vi "bulk_read_write.vi"() -> ()   [LabVIEW 2022 SP3]
uses:
  Library/dxl_x64_c.lvlib
panel:
  out "dynamixel_error":string
  out "dynamixel_comm_result":string
  in  "value : PRO (slide)\nLED RED":bool
  in  "LEN_PRO_\nGOAL_POSITION":u16=4
  out "groupwrite_num":i32
  in  "LEN_PRO_\nLED_RED":u16=1
  in  "ADDR_PRO_\nLED_RED":u16=563
  out "value : PRO (LED)\nLED_RED":bool
  out "groupread_num":i32
  in  "LEN_PRO_\nPRESENT_POSITION":u16=4
  in  "dynamixe2_id":u8=2
  in  "device_name":string="COM1"
  in  "ADDR_PRO_\nPRESENT_POSITION":u16=611
  in  "ADDR_PRO_\nGOAL_POSITION":u16=596
  in  "ADDR_PRO_\nTORQUE_ENABLE":u16=562
  out "protocol_version":dbl=2.0
  out "value : PRO (knob)\npresent position 1":i32(knob) scale=150000.0..-150000.0
  in  "terminate":bool
  out "port_num":i32
  in  "value : PRO (dial)\ngoal position":i32(knob) scale=150000.0..-150000.0
  in  "dynamixel1_id":u8=1
  in  "baud_rate":i32=57600
  # "/*******************************************************************************\n* Copyright (c) 2016, ROBOTIS CO., LTD.\n* All rights reserved.\n*\n* Redistribution and use in source and binary forms, with or without\n* modification, are permitted provided that the following conditions are met:\n*\n* * Redistributions of source code must retain the above copyright notice, this\n*   list of conditions and the following disclaimer.\n*\n* * Redistributions in binary form must reproduce the above copyright notice,\n*   this list of conditions and the following disclaimer in the documentation\n*   and/or other materials provided with the distribution.\n*\n* * Neither the name of ROBOTIS nor the names of its\n*   contributors may be used to endorse or promote products derived from\n*   this software without specific prior written permission.\n*\n* THIS SOFTWARE IS PROVIDED BY THE COPYRIGHT HOLDERS AND CONTRIBUTORS \"AS IS\"\n* AND ANY EXPRESS OR IMPLIED WARRANTIES, INCLUDING, BUT NOT LIMITED TO, THE\n* IMPLIED WARRANTIES OF MERCHANTABILITY AND FITNESS FOR A PARTICULAR PURPOSE ARE\n* DISCLAIMED. IN NO EVENT SHALL THE COPYRIGHT HOLDER OR CONTRIBUTORS BE LIABLE\n* FOR ANY DIRECT, INDIRECT, INCIDENTAL, SPECIAL, EXEMPLARY, OR CONSEQUENTIAL\n* DAMAGES (INCLUDING, BUT NOT LIMITED TO, PROCUREMENT OF SUBSTITUTE GOODS OR\n* SERVICES; LOSS OF USE, DATA, OR PROFITS; OR BUSINESS INTERRUPTION) HOWEVER\n* CAUSED AND ON ANY THEORY OF LIABILITY, WHETHER IN CONTRACT, STRICT LIABILITY,\n* OR TORT (INCLUDING NEGLIGENCE OR OTHERWISE) ARISING IN ANY WAY OUT OF THE USE\n* OF THIS SOFTWARE, EVEN IF ADVISED OF THE POSSIBILITY OF SUCH DAMAGE.\n*******************************************************************************/\n\n/* Author: Ryu Woon Jung (Leon) */"
  # "Available Dynamixel model on this example : All models using Protocol 2.0\nThis example is designed for using two Dynamixel PRO 54-200, and an USB2DYNAMIXEL.\nTo use another Dynamixel model, such as X series, see their details in E-Manual(support.robotis.com) \n   and edit \"numeric control\"s seen left with \"Edit Text\" tool.\nBe sure that Dynamixel PRO properties are already set as %% ID : 1 / Baudnum : 1 (Baudrate : 57600)\n\n1. Run example by click above \"Run\" button (below \"Edit\" menu).\n2. Drag \"dial\" then you may see the Dynamixel and \"knob\"s rotating\n3. Click \"slide button\" then you may see the LED of Dynamixel lighting\n4. To finish the example, press \"terminate\" button."
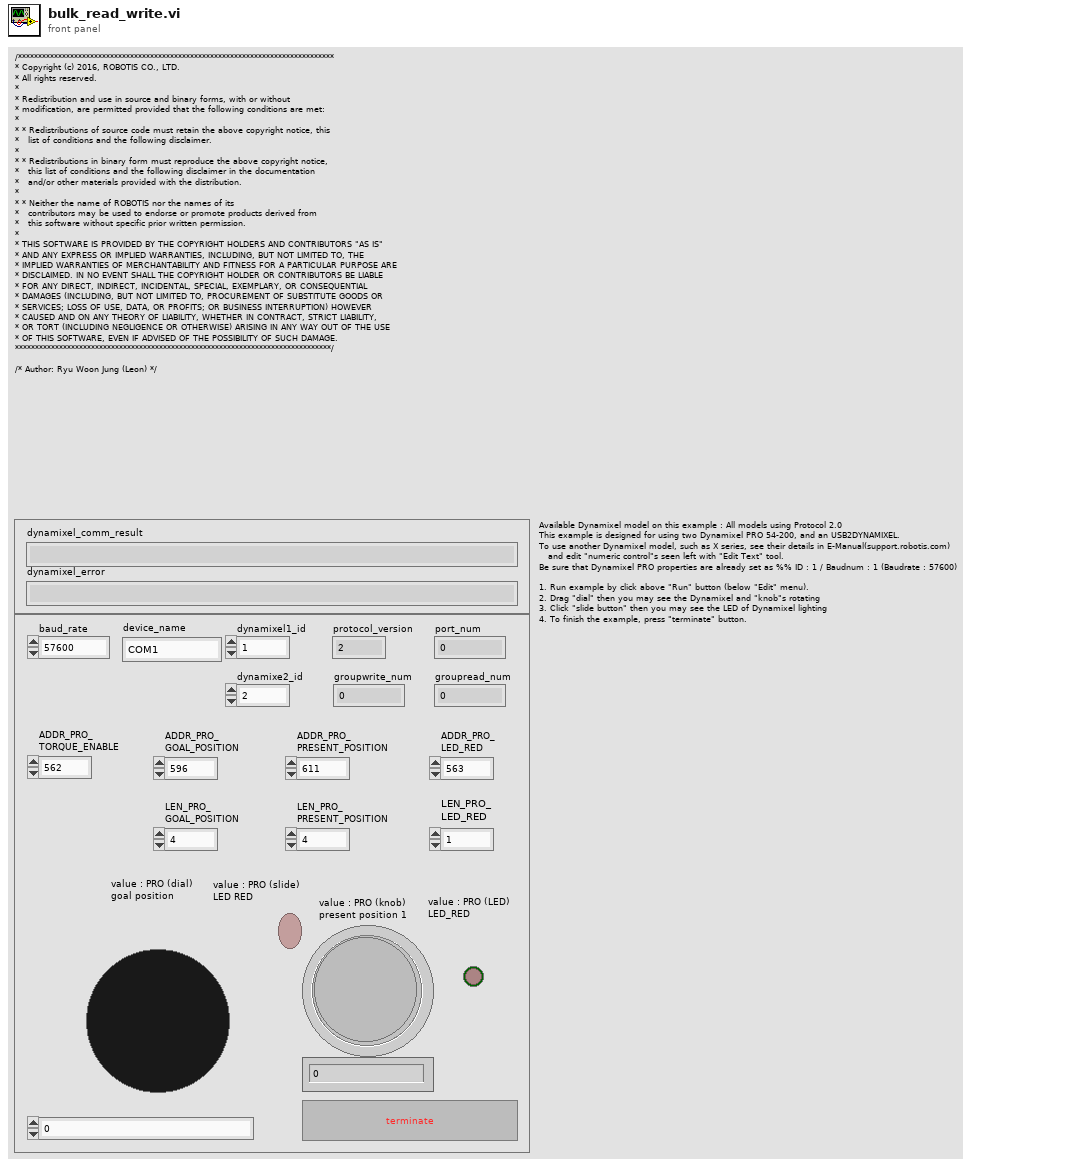
[diagram p1: front panel]
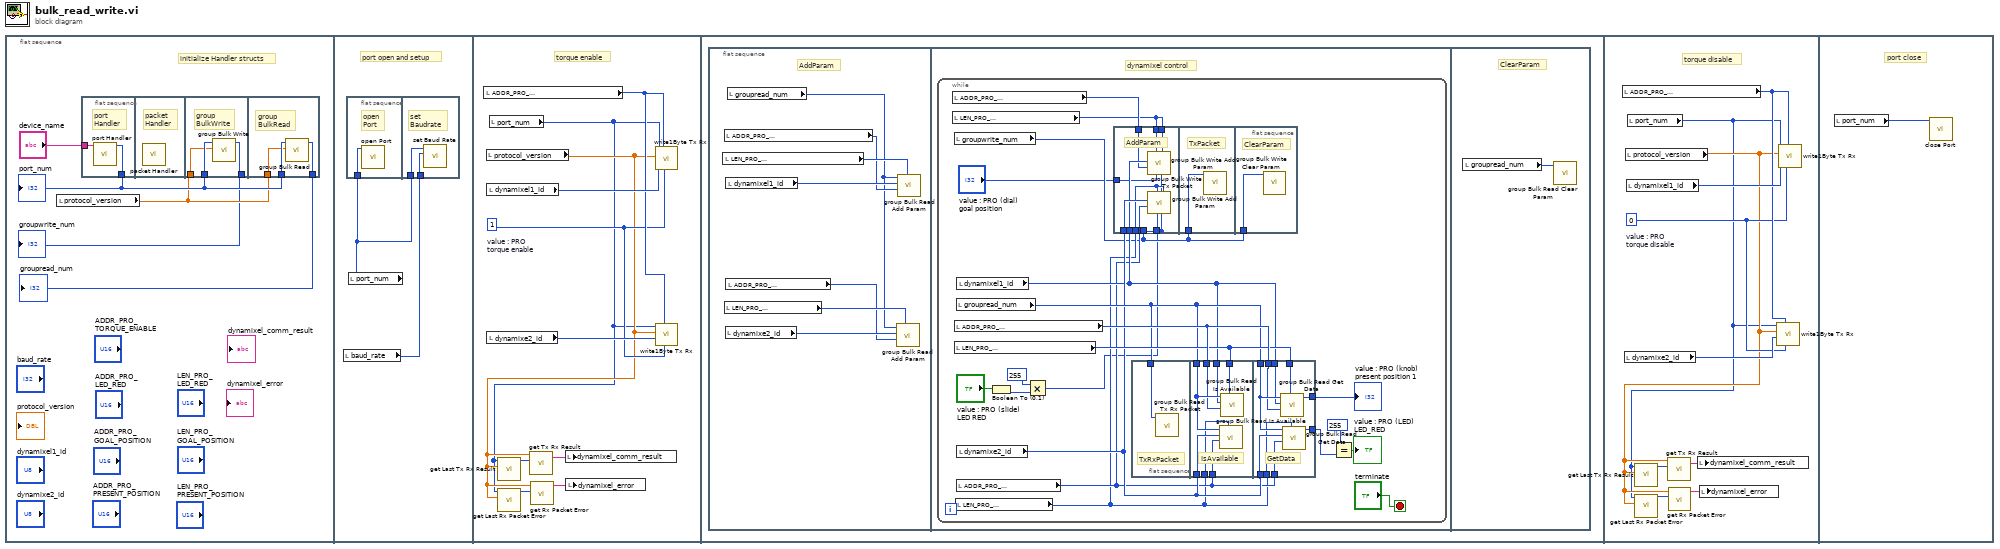
[diagram p0: block diagram]
diagram:
  n1 = flat-sequence {
    frame #0 {
      # "initialize Handler structs"
      n2 = local read "protocol_version"() -> (w3:dbl)
      n3 = flat-sequence {
        tunnel: "device_name" -> [w7]
        tunnel: [w6] -> w4
        tunnel: w3 -> [w8]
        tunnel: w4 -> [w10]
        tunnel: [w9] -> w2
        tunnel: w4 -> [w13]
        tunnel: w3 -> [w12]
        tunnel: [w11] -> w1
        frame #0 {
          # "port\nHandler"
          n4 = call "port Handler.vi"("port_name"=w7) -> ("function return"=w6:i32)  [unwired: 9 in, 1 out]
        }
        frame #1 {
          # "packet\nHandler"
          n5 = call "packet Handler.vi"() -> ()  [unwired: 11 in, 1 out]
        }
        frame #2 {
          # "group\nBulkWrite"
          n6 = call "group Bulk Write.vi"("protocol_version"=w8, "port_num"=w10) -> ("function return"=w9:i32)  [unwired: 8 in, 1 out]
        }
        frame #3 {
          # "group\nBulkRead"
          n7 = call "group Bulk Read.vi"("protocol_version"=w12, "port_num"=w13) -> ("function return"=w11:i32)  [unwired: 8 in, 1 out]
        }
      }
      "port_num" <- w4
      "groupread_num" <- w1
      "groupwrite_num" <- w2
    }
    frame #1 {
      # "port open and setup"
      n8 = local read "baud_rate"() -> (w14:i32)
      n9 = flat-sequence {
        tunnel: w15 -> [w16]
        tunnel: w15 -> [w18]
        tunnel: w14 -> [w17]
        frame #0 {
          # "open\nPort"
          n10 = call "open Port.vi"("port_num"=w16) -> ()  [unwired: 9 in, 2 out]
        }
        frame #1 {
          # "set\nBaudrate"
          n11 = call "set Baud Rate.vi"("baudrate"=w17, "port_num"=w18) -> ()  [unwired: 8 in, 2 out]
        }
      }
      n12 = local read "port_num"() -> (w15:i32)
    }
    frame #2 {
      w25 = 1  # value : PRO torque enable
      # "torque enable"
      n13 = local read "ADDR_PRO_\nTORQUE_ENABLE"() -> (w27:u16)
      n14 = local read "protocol_version"() -> (w20:dbl)
      n15 = local read "dynamixel1_id"() -> (w28:u8)
      n16 = local read "dynamixe2_id"() -> (w26:u8)
      n17 = local read "port_num"() -> (w19:i32)
      n18 = call "get Last Tx Rx Result.vi"("protocol_version"=w20, "port_num"=w19) -> ("function return"=w21:i32)  [unwired: 8 in, 1 out]
      n19 = call "get Last Rx Packet Error.vi"("protocol_version"=w20, "port_num"=w19) -> ("function return"=w22:u8)  [unwired: 8 in, 1 out]
      n20 = call "get Tx Rx Result.vi"("result"=w21, "protocol_version"=w20) -> ("function return"=w24:string)  [unwired: 8 in, 1 out]
      n21 = call "get Rx Packet Error.vi"("error"=w22, "protocol_version"=w20) -> ("function return"=w23:string)  [unwired: 8 in, 1 out]
      n22 = local write "dynamixel_comm_result"(w24) -> ()
      n23 = local write "dynamixel_error"(w23) -> ()
      n24 = call "write1Byte Tx Rx.vi"("data"=w25, "address"=w27, "id"=w28, "protocol_version"=w20, "port_num"=w19) -> ()  [unwired: 6 in, 1 out]
      n25 = call "write1Byte Tx Rx.vi"("data"=w25, "address"=w27, "id"=w26, "protocol_version"=w20, "port_num"=w19) -> ()  [unwired: 6 in, 1 out]
    }
    frame #3 {
      n26 = flat-sequence {
        frame #0 {
          # "AddParam"
          n27 = local read "LEN_PRO_\nPRESENT_POSITION"() -> (w35:u16)
          n28 = local read "ADDR_PRO_\nPRESENT_POSITION"() -> (w33:u16)
          n29 = local read "LEN_PRO_\nLED_RED"() -> (w32:u16)
          n30 = local read "dynamixe2_id"() -> (w30:u8)
          n31 = local read "dynamixel1_id"() -> (w34:u8)
          n32 = local read "ADDR_PRO_\nLED_RED"() -> (w29:u16)
          n33 = local read "groupread_num"() -> (w31:i32)
          n34 = call "group Bulk Read Add Param.vi"("data_length"=w32, "start_address"=w29, "id"=w30, "group_num"=w31) -> ()  [unwired: 6 in, 2 out]
          n35 = call "group Bulk Read Add Param.vi"("data_length"=w35, "start_address"=w33, "id"=w34, "group_num"=w31) -> ()  [unwired: 6 in, 2 out]
        }
        frame #1 {
          # "dynamixel control"
          n36 = while {
            stop <- "terminate" stop-if-true
            n37 = local read "ADDR_PRO_\nGOAL_POSITION"() -> (w44:u16)
            n38 = local read "LEN_PRO_\nGOAL_POSITION"() -> (w43:u16)
            n39 = local read "groupwrite_num"() -> (w41:i32)
            n40 = local read "ADDR_PRO_\nPRESENT_POSITION"() -> (w54:u16)
            n41 = local read "LEN_PRO_\nPRESENT_POSITION"() -> (w50:u16)
            n42 = local read "LEN_PRO_\nLED_RED"() -> (w45:u16)
            n43 = local read "groupread_num"() -> (w49:i32)
            n44 = local read "ADDR_PRO_\nLED_RED"() -> (w46:u16)
            n45 = local read "dynamixel1_id"() -> (w47:u8)
            n46 = local read "dynamixe2_id"() -> (w48:u8)
            n47 = Boolean To (0,1)(Boolean="value : PRO (slide)\nLED RED") -> (0, 1=w38:i16)
            n48 = Multiply(x=255, y=w38) -> (x*y=w37:i32)
            n49 = flat-sequence {
              tunnel: [w56] -> _
              tunnel: w48 -> [w65]
              tunnel: w47 -> [w64]
              tunnel: w46 -> [w63]
              tunnel: w45 -> [w59]
              tunnel: w44 -> [w62]
              tunnel: w43 -> [w61]
              tunnel: w43 -> [w60]
              tunnel: "value : PRO (dial)\ngoal position" -> [w58]
              tunnel: w37 -> [w57]
              tunnel: w41 -> [w56]
              tunnel: w41 -> [w66]
              tunnel: w41 -> [w67]
              frame #0 {
                # "AddParam"
                n50 = call "group Bulk Write Add Param.vi"("input_length"=w60, "data"=w58, "data_length"=w61, "start_address"=w62, "id"=w64, "group_num"=w56) -> ()  [unwired: 4 in, 2 out]
                n51 = call "group Bulk Write Add Param.vi"("input_length"=w59, "data"=w57, "data_length"=w59, "start_address"=w63, "id"=w65, "group_num"=w56) -> ()  [unwired: 4 in, 2 out]
              }
              frame #1 {
                # "TxPacket"
                n52 = call "group Bulk Write Tx Packet.vi"("group_num"=w66) -> ()  [unwired: 10 in, 1 out]
              }
              frame #2 {
                # "ClearParam"
                n53 = call "group Bulk Write Clear Param.vi"("group_num"=w67) -> ()  [unwired: 10 in, 1 out]
              }
            }
            n54 = flat-sequence {
              tunnel: w49 -> [w68]
              tunnel: w49 -> [w75]
              tunnel: w48 -> [w74]
              tunnel: w54 -> [w73]
              tunnel: w45 -> [w72]
              tunnel: w46 -> [w71]
              tunnel: w50 -> [w70]
              tunnel: w47 -> [w69]
              tunnel: w49 -> [w84]
              tunnel: w48 -> [w83]
              tunnel: w54 -> [w82]
              tunnel: w45 -> [w79]
              tunnel: [w81] -> w39
              tunnel: [w80] -> w51
              tunnel: w46 -> [w78]
              tunnel: w50 -> [w77]
              tunnel: w47 -> [w76]
              frame #0 {
                # "TxRxPacket"
                n55 = call "group Bulk Read Tx Rx Packet.vi"("group_num"=w68) -> ()  [unwired: 10 in, 1 out]
              }
              frame #1 {
                # "IsAvailable"
                n56 = call "group Bulk Read Is Available.vi"("data_length"=w72, "address"=w71, "id"=w74, "group_num"=w75) -> ()  [unwired: 6 in, 2 out]
                n57 = call "group Bulk Read Is Available.vi"("data_length"=w70, "address"=w73, "id"=w69, "group_num"=w75) -> ()  [unwired: 6 in, 2 out]
              }
              frame #2 {
                # "GetData"
                n58 = call "group Bulk Read Get Data.vi"("data_length"=w77, "address"=w82, "id"=w76, "group_num"=w84) -> ("function return"=w80:u32)  [unwired: 6 in, 1 out]
                n59 = call "group Bulk Read Get Data.vi"("data_length"=w79, "address"=w78, "id"=w83, "group_num"=w84) -> ("function return"=w81:u32)  [unwired: 6 in, 1 out]
              }
            }
            n60 = Equal?(x=255, y=w39) -> (x = y?=→"value : PRO (LED)\nLED_RED":bool)
            "value : PRO (knob)\npresent position 1" <- w51
          }
        }
        frame #2 {
          # "ClearParam"
          n61 = local read "groupread_num"() -> (w85:i32)
          n62 = call "group Bulk Read Clear Param.vi"("group_num"=w85) -> ()  [unwired: 10 in, 1 out]
        }
      }
    }
    frame #4 {
      w92 = 0  # value : PRO torque disable
      # "torque disable"
      n63 = local read "ADDR_PRO_\nTORQUE_ENABLE"() -> (w94:u16)
      n64 = local read "dynamixe2_id"() -> (w93:u8)
      n65 = local read "protocol_version"() -> (w87:dbl)
      n66 = local read "dynamixel1_id"() -> (w95:u8)
      n67 = local read "port_num"() -> (w86:i32)
      n68 = call "get Last Tx Rx Result.vi"("protocol_version"=w87, "port_num"=w86) -> ("function return"=w89:i32)  [unwired: 8 in, 1 out]
      n69 = call "get Last Rx Packet Error.vi"("protocol_version"=w87, "port_num"=w86) -> ("function return"=w88:u8)  [unwired: 8 in, 1 out]
      n70 = call "get Tx Rx Result.vi"("result"=w89, "protocol_version"=w87) -> ("function return"=w90:string)  [unwired: 8 in, 1 out]
      n71 = call "get Rx Packet Error.vi"("error"=w88, "protocol_version"=w87) -> ("function return"=w91:string)  [unwired: 8 in, 1 out]
      n72 = local write "dynamixel_comm_result"(w90) -> ()
      n73 = local write "dynamixel_error"(w91) -> ()
      n74 = call "write1Byte Tx Rx.vi"("data"=w92, "address"=w94, "id"=w93, "protocol_version"=w87, "port_num"=w86) -> ()  [unwired: 6 in, 1 out]
      n75 = call "write1Byte Tx Rx.vi"("data"=w92, "address"=w94, "id"=w95, "protocol_version"=w87, "port_num"=w86) -> ()  [unwired: 6 in, 1 out]
    }
    frame #5 {
      # "port close"
      n76 = local read "port_num"() -> (w96:i32)
      n77 = call "close Port.vi"("port_num"=w96) -> ()  [unwired: 10 in, 1 out]
    }
  }
